vi "Dvmg Get Dev Type.vi"(8 "error in (no error)":errorcluster, 9 "perc":i32, 10 "dvtp":i32, 11 "idvc":i32) -> (0 "error out":errorcluster, 1 "perc out":i32, 2 "dvtp out":i32, 3 "function return":i32)   [LabVIEW 2011, in "LVH-Adept.lvlib" / "DPCUTIL.lvlib"]
doc: "DPCAPI BOOL DvmgGetDevType(INT32 idvc, INT32 * dvtp, ERC * perc);"
uses:
  DPCUTIL.lvlib
  dpcutil.dll
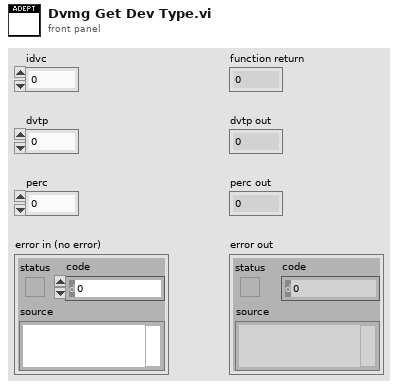
[diagram p1: front panel]
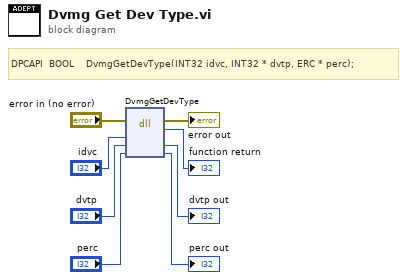
[diagram p0: block diagram]
diagram:
  # "DPCAPI  BOOL    DvmgGetDevType(INT32 idvc, INT32 * dvtp, ERC * perc);"
  n1 = dll-call lib="dpcutil.*" fn="DvmgGetDevType"(error in="error in (no error)", "idvc"="idvc", "dvtp"="dvtp", "perc"="perc") -> (error out=→"error out":errorcluster, →"function return":i32, "dvtp"=→"dvtp out":i32, "perc"=→"perc out":i32)  [unwired: 3 in, 1 out]
